vi "Wait for State.vi"(8 "error in":errorcluster, 9 "timeout in ms":i32=20, 10 "expected states":T1[](array[typedef]), 11 "Standard Engine in":refnum<class "Standard Engine Runtime.lvclass">) -> (0 "error out":errorcluster, 3 "Standard Engine out":refnum<class "Standard Engine Runtime.lvclass">)   [LabVIEW 2013, in "Standard Engine Runtime.lvclass"]
uses:
  Standard Engine Runtime.lvclass
  <vilib>/NI/Module Execution Interface/Engine Runtime/Execution States.ctl
  Standard Engine Runtime.lvclass/Standard Engine Runtime.ctl
  <vilib>/NI/Module Execution Interface/Engine Runtime/Engine Runtime Interface.lvclass
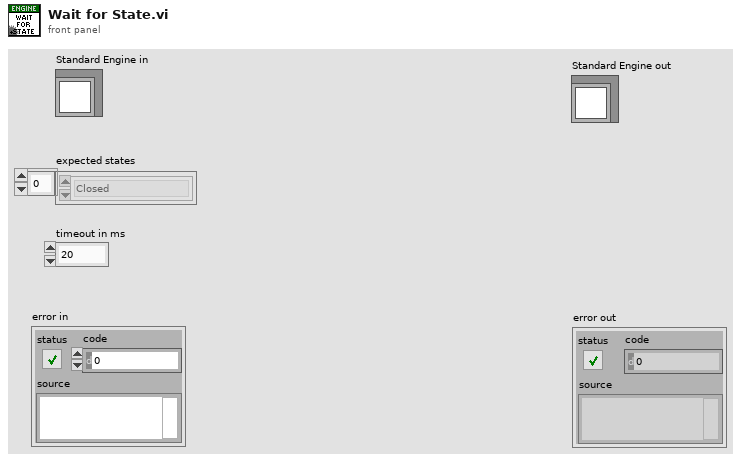
[diagram p1: front panel]
types:
  T1 = typedef "Engine Runtime Interface.lvclass/Execution States.ctl" = enum16{"Initializing", "Paused (Initialized)", "Running", "Set Safe Outputs", "Uninitializing", "Stopped (Uninitialized)", "Error (Uninitialized)", "Safe State (Uninitialized)", "Closed"}
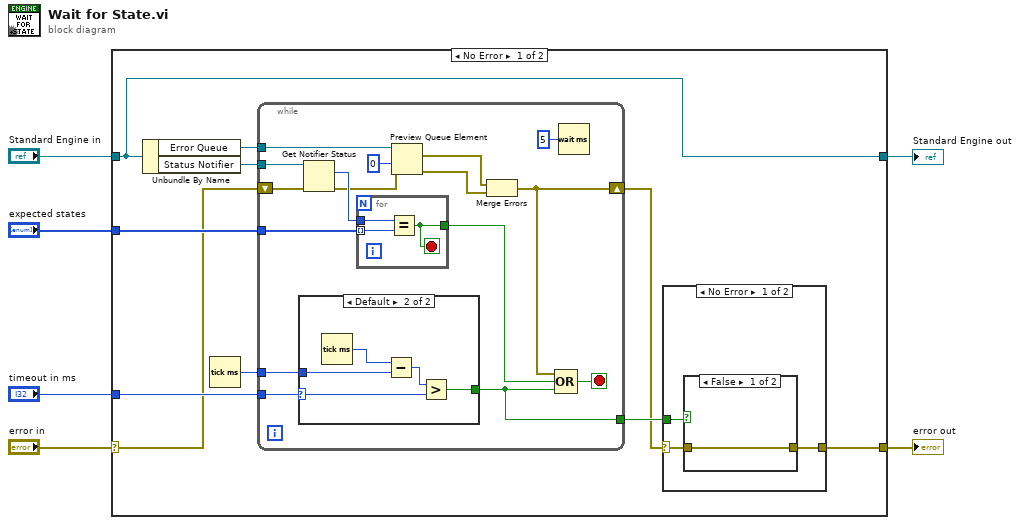
[diagram p0: block diagram]
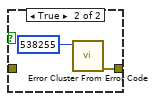
[diagram p2: hidden frame]
diagram:
  n1 = case shown="No Error" "error in" {
    selector: "error in" -> [w13 w49]
    tunnel: [w11 w49] -> w6
    tunnel: "timeout in ms" -> [w16 _]
    tunnel: "expected states" -> [w14 _]
    tunnel: "Standard Engine in" -> [w9 w48]
    tunnel: [w9 w48] -> w1
    frame No Error {
      n2 = Unbundle By Name(w9) -> ("Error Queue"=w8:refnum<queue>, "Status Notifier"=w10:refnum<notifier>)
      n3 = Tick Count (ms)() -> (millisecond timer value=w15:u32)
      n4 = while {
        tunnel: w10 -> [w39]
        tunnel: w16 -> [w30]
        tunnel: w15 -> [w36]
        tunnel: w14 -> [w35]
        tunnel: [w31] -> w12
        tunnel: w8 -> [w29]
        shift-right: [w24] -> w7
        shift-left: w13 -> [w38]
        stop <- w32 stop-if-true
        n5 = case shown="Default" w30 {
          selector: w30 -> [_ w40]
          tunnel: w36 -> [_ w43]
          tunnel: [_ w41] -> w31
          frame -1 {
            # "-1 means never timeout"
          }
          frame Default {
            n6 = Tick Count (ms)() -> (millisecond timer value=w44:u32)
            n7 = Subtract(x=w44, y=w43) -> (x-y=w42:u32)
            n8 = Greater?(x=w42, y=w40) -> (0:w41:bool)
          }
        }
        n9 = Get Notifier Status(notifier=w39, error in (no error)=w38) -> (current notification=w34:T1, error out=w28:errorcluster)  [unwired: 3 out]
        n10 = for {
          tunnel: w35 -> [w46] mode=indexing
          tunnel: w34 -> [w47]
          tunnel: [w45] -> w33
          stop <- w45 stop-if-true
          n11 = Equal?(x=w47, y=w46) -> (x = y?=w45:bool)
        }
        n12 = Preview Queue Element(queue=w29, timeout in ms (-1)=0, error in (no error)=w28) -> (element=w25:errorcluster, error out=w26:errorcluster)  [unwired: 2 out]
        n13 = Merge Errors(w25, w26) -> (w24:errorcluster)
        n14 = Compound Arithmetic op=OR(w24, w33, w31) -> (w32:bool)
        n15 = Wait (ms)(milliseconds to wait=u32 5) -> ()  [unwired: 1 out]
      }
      n16 = case shown="No Error" w7 {
        selector: w7 -> [w17 w23]
        tunnel: w12 -> [w18 _]
        tunnel: [w19 w23] -> w11
        frame No Error {
          n17 = case shown="False" w18 {
            tunnel: [w20 w21] -> w19
            tunnel: w17 -> [w20 _]
            frame False {
            }
            frame True {
              n18 = call <vilib>:"Error Cluster From Error Code.vi"("error code (0)"=538255) -> ("error out"=w21:errorcluster)  [unwired: 8 in]
            }
          }
        }
        frame Error {
        }
      }
    }
    frame Error {
    }
  }
  "error out" <- w6
  "Standard Engine out" <- w1
